vi "CreateVIWrapper.vi"(8 "error in (no error)":errorcluster, 9 "Method Help":string, 10 "Method Name":string) -> (0 "error out":errorcluster, 2 "VI Path":path)   [LabVIEW 2017, in "WebServiceImporter.lvlib" / "VI Generator.lvlib"]
doc: "Create one wrapper VI for a method in assembly given by 'Proxy DLL Location'. 'Method Name' si the qualified name of the method( class.method )"
uses:
  <vilib>/Platform/WebService/VI Generator/VI Generator.lvlib
  <vilib>/Platform/WebService/Error Handling/Error/Error Number.ctl
  <vilib>/Platform/WebService/Error Handling/Error/Context Name.ctl
  <vilib>/Platform/WebService/Error Handling/Error Handling.lvlib
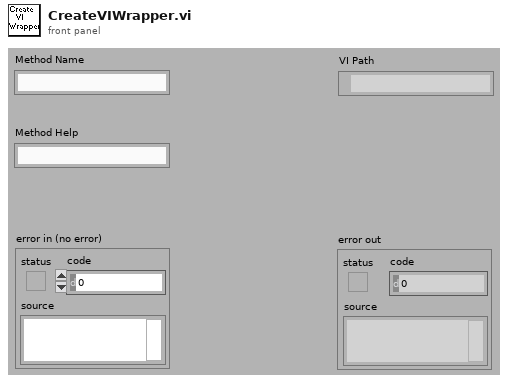
[diagram p1: front panel]
types:
  T1 = typedef "WebServiceImporter.lvlib/Error Handling.lvlib/Context Name.ctl" = u16
  T2 = typedef "WebServiceImporter.lvlib/Error Handling.lvlib/Error Number.ctl" = u16
  T3 = typedef "WebServiceImporter.lvlib/Error Handling.lvlib/Context.ctl" = cluster{"name":T1, "value":string}[]
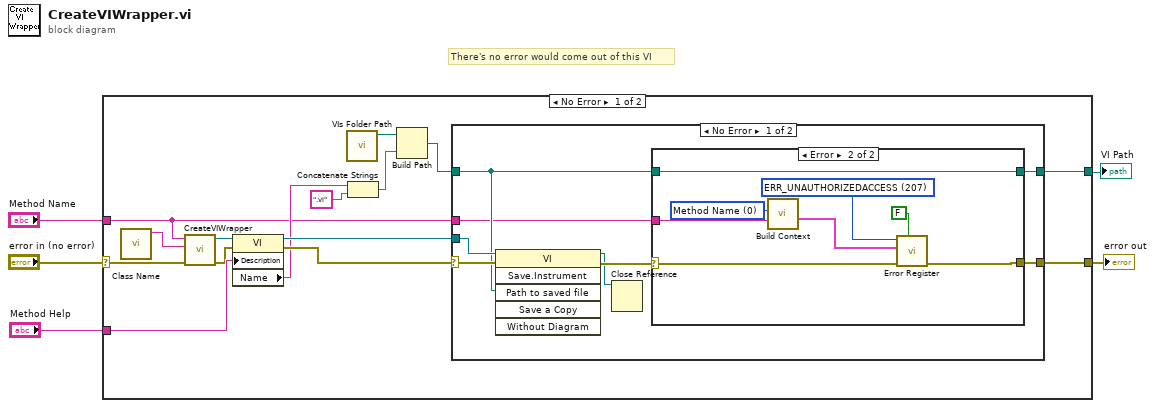
[diagram p0: block diagram]
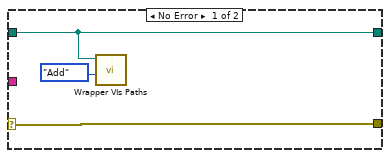
[diagram p2: hidden frame]
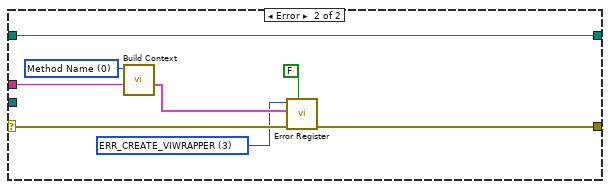
[diagram p3: hidden frame]
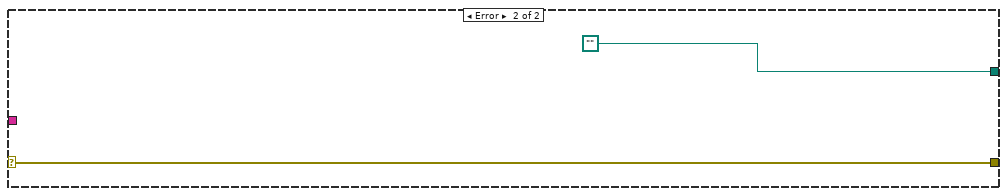
[diagram p4: hidden frame]
diagram:
  # "There's no error would come out of this VI"
  n1 = case shown="No Error" "error in (no error)" {
    selector: "error in (no error)" -> [w10 w48]
    tunnel: "Method Name" -> [w6 _]
    tunnel: [w18 w48] -> w3
    tunnel: [w16 path ""] -> w2
    tunnel: "Method Help" -> [w12 _]
    frame No Error {
      n2 = call <vilib>:"Class Name.vi"() -> ("Class Name (out)"=w7:string)  [unwired: 3 in, 8 out]
      n3 = call <vilib>:"CreateVIWrapper.vi"("error in (no error)"=w10, "Class Name"=w7, "Method Name"=w6) -> ("error out"=w8:errorcluster, "VI Reference Out"=w9:refnum<vi>)  [unwired: 7 out]
      n4 = property class="VI"(reference=w9, error in=w8, "Description"=w12) -> (reference out=w14:refnum<vi>, error out=w13:errorcluster, "Name"=w11:string)
      n5 = call <vilib>:"VIs Folder Path.vi"() -> ("Path 2"=w15:path)  [unwired: 3 in, 8 out]
      n6 = Concatenate Strings(w11, ".vi" ("string")) -> (w20:string)
      n7 = Build Path(base path=w15, name or relative path=w20) -> (appended path=w17:path)
      n8 = case shown="No Error" w13 {
        selector: w13 -> [w27 w44]
        tunnel: w14 -> [w28 _]
        tunnel: [w25 w43] -> w18
        tunnel: w17 -> [w26 w40]
        tunnel: w6 -> [w21 w47]
        tunnel: [w24 w40] -> w16
        frame No Error {
          n9 = invoke class="VI" method="Save.Instrument"(reference=w28, error in=w27, "Path to saved file"=w26) -> (reference out=w22:refnum<vi>, error out=w23:errorcluster)  [unwired: 3 in, 4 out]
          n10 = Close Reference(reference=w22) -> ()  [unwired: 1 in, 1 out]
          n11 = case shown="Error" w23 {
            selector: w23 -> [w30 w35]
            tunnel: w26 -> [w29 w39]
            tunnel: [w30 w34] -> w25
            tunnel: [w29 w39] -> w24
            tunnel: w21 -> [_ w32]
            frame No Error {
              n12 = call <vilib>:"Wrapper VIs Paths.vi"("Op"=enum16{"Get", "Add", "Clear"}."Add", "Path"=w29) -> ()  [unwired: 1 in, 9 out]
            }
            frame Error {
              w33 = T1 0 items=["Method Name", "Parameter Name", "VI Name", "Control Name", "Proxy Dll Path", "Project Library Name"] ("Context Name")
              w36 = T2 207 items=["ERR_NOERROR"=0, "ERR_ACCESS_OUTPUTFOLDER"=1, "ERR_INVALID_LIBRARYNAME"=2, "ERR_CREATE_VIWRAPPER"=3, "ERR_UNKNOWN"=201, "ERR_BAD_ARGUMENT"=202, "ERR_URL_NOTFOUND_BADWSDL"=203, "ERR_BADLYFORMATTEDURL"=204, "ERR_BADHOSTNAME"=205, "ERR_BADDIRECTORY"=206, "ERR_UNAUTHORIZEDACCESS"=207] ("Error Number")
              n13 = call <vilib>:"Build Context.vi"("Context Value"=w32, "Context Name"=w33) -> ("Context"=w37:T3)  [unwired: 9 out]
              n14 = call <vilib>:"Error Register.vi"("Throw Up?"=FALSE, "error in (no error)"=w35, "Context"=w37, "Error Number"=w36) -> ("error out"=w34:errorcluster)  [unwired: 1 in, 6 out]
            }
          }
        }
        frame Error {
          w41 = T2 3 items=["ERR_NOERROR"=0, "ERR_ACCESS_OUTPUTFOLDER"=1, "ERR_INVALID_LIBRARYNAME"=2, "ERR_CREATE_VIWRAPPER"=3, "ERR_UNKNOWN"=201, "ERR_BAD_ARGUMENT"=202, "ERR_URL_NOTFOUND_BADWSDL"=203, "ERR_BADLYFORMATTEDURL"=204, "ERR_BADHOSTNAME"=205, "ERR_BADDIRECTORY"=206, "ERR_UNAUTHORIZEDACCESS"=207] ("Error Number")
          w46 = T1 0 items=["Method Name", "Parameter Name", "VI Name", "Control Name", "Proxy Dll Path"] ("Context Name")
          n15 = call <vilib>:"Build Context.vi"("Context Value"=w47, "Context Name"=w46) -> ("Context"=w42:T3)  [unwired: 9 out]
          n16 = call <vilib>:"Error Register.vi"("Throw Up?"=FALSE, "error in (no error)"=w44, "Context"=w42, "Error Number"=w41) -> ("error out"=w43:errorcluster)  [unwired: 1 in, 6 out]
        }
      }
    }
    frame Error {
    }
  }
  "VI Path" <- w2
  "error out" <- w3
